vi "I2C Close Channel.vi"(0 "handle":u32, 11 "error in (no error)":errorcluster) -> (15 "error out":errorcluster)   [LabVIEW 2017, in "libMPSSE.lvlib"]
doc: "FTDI_API FT_STATUS I2C_CloseChannel(FT_HANDLE handle);"
uses:
  libMPSSE.lvlib
  libMPSSE-SPI-LabVIEW-master/libMPSSE.dll
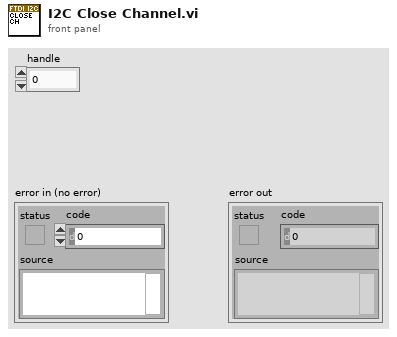
[diagram p1: front panel]
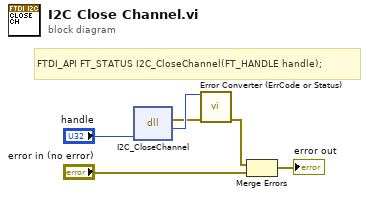
[diagram p0: block diagram]
diagram:
  # "FTDI_API FT_STATUS I2C_CloseChannel(FT_HANDLE handle);"
  n1 = dll-call lib="\\\\Mac\\Home/Desktop/libMPSSE-SPI-LabVIEW-master/libMPSSE.dll" fn="I2C_CloseChannel"("handle"="handle") -> (error out=w4:errorcluster, "return type"=w6:u32)  [unwired: 4 in, 1 out]
  n2 = call "Error Converter (ErrCode or Status).vi"("error code"=w6, "error in (no error)"=w4) -> ("error out"=w2:errorcluster)  [unwired: 13 in]
  n3 = Merge Errors(w2, "error in (no error)") -> (→"error out":errorcluster)
